vi "Create Element Array.vi"(8 "error in (no error)":errorcluster, 10 "Length value (auto)":string, 11 "Contents":refnum<class "Data Item.lvclass">[](array[class])) -> (0 "error out":errorcluster, 3 "Element Array":refnum<class "Element Array.lvclass">)   [LabVIEW 2020, in "VILab.lvlib" / "Element Array.lvclass"]
uses:
  Element Array.lvclass
  Data Item/Data Item.lvclass
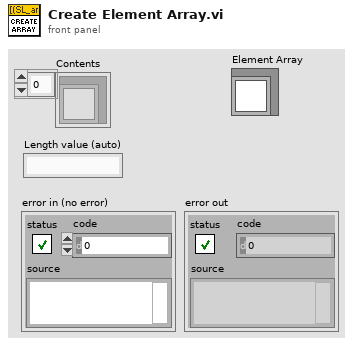
[diagram p1: front panel]
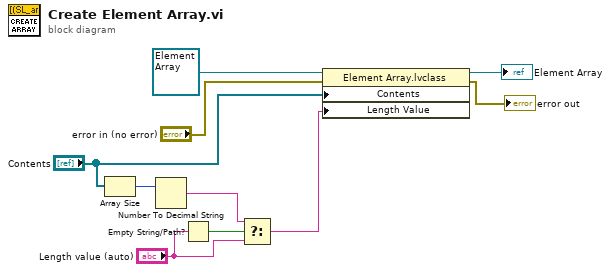
[diagram p0: block diagram]
diagram:
  n1 = Array Size(array="Contents") -> (size(s)=w3:i32)
  n2 = Number To Decimal String(number=w3) -> (decimal integer string=w2:string)  [unwired: 1 in]
  n3 = Empty String/Path?(string/path="Length value (auto)") -> (empty?=w6:bool)
  n4 = Select(t=w2, s=w6, f="Length value (auto)") -> (s? t:f=w1:string)
  n5 = property class="Element Array.lvclass"(reference=refnum<class "Element Array.lvclass"> refnum ("VILab.lvlib:Element Array.lvclass"), error in="error in (no error)", "Contents"="Contents", "Length Value"=w1) -> (reference out=→"Element Array":refnum<class "Element Array.lvclass">, error out=→"error out":errorcluster)
